vi "Short-Term Flicker Severity.vi"(0 "Pinst":waveform(dbl)[](array[waveform]), 1 "reset? (F)":bool, 9 "system info in":refnum<class "EP System Info.lvclass">, 11 "error in (no error)":errorcluster) -> (4 "Pst":dbl[](array[numeric]), 6 "Pst timestamp":timestamp, 10 "system info out":refnum<class "EP System Info.lvclass">, 14 "output valid?":bool, 15 "error out":errorcluster)   [LabVIEW 2014, in "NI_EP_Power Quality.lvlib"]
doc: "Aggregates instantaneous flicker values and returns the short-term flicker of a voltage waveform for a 10-minute period, according to IEC 61000-4-15:2010.\n\nThis VI supports measuring single-bus single-line or multiple-bus single-line systems."
uses:
  <vilib>/addons/Electrical Power/PQ/NI_EP_Power Quality.lvlib
  <vilib>/addons/Electrical Power/PQ/Common/Classes/System Info/EP System Info.lvclass
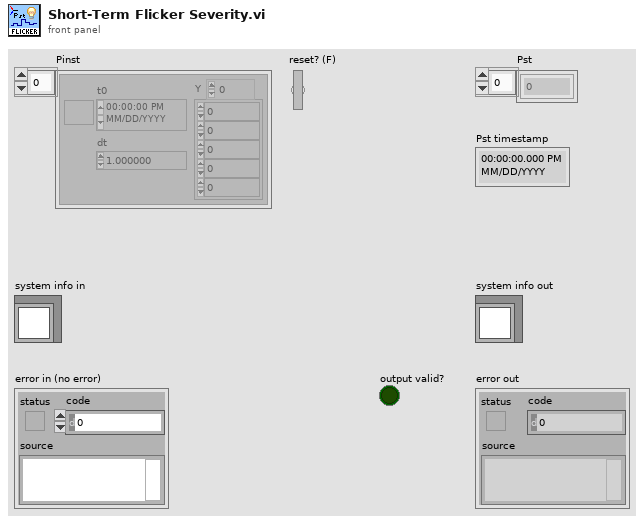
[diagram p1: front panel]
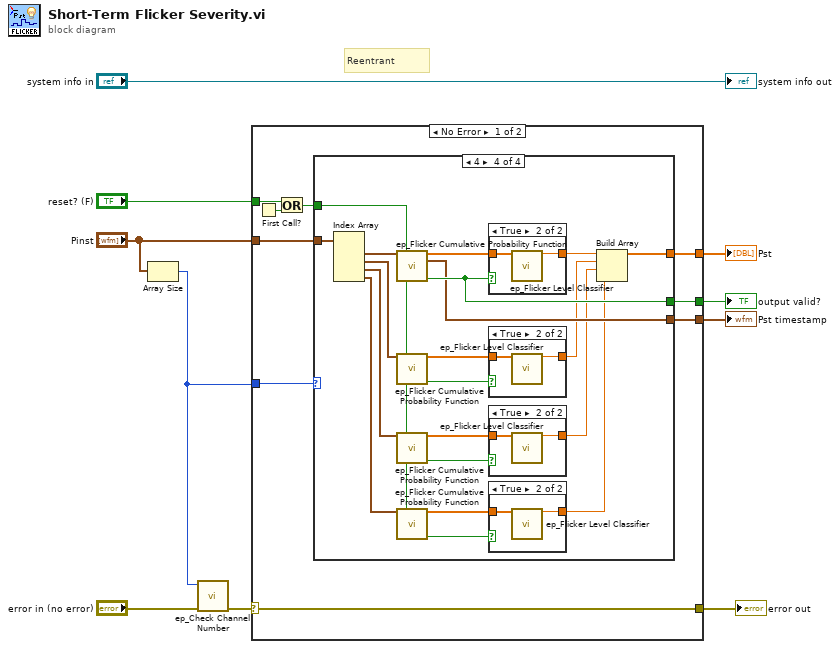
[diagram p0: block diagram]
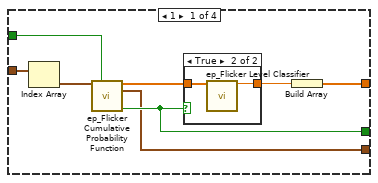
[diagram p2: hidden frame]
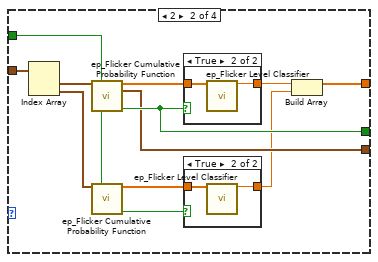
[diagram p4: hidden frame]
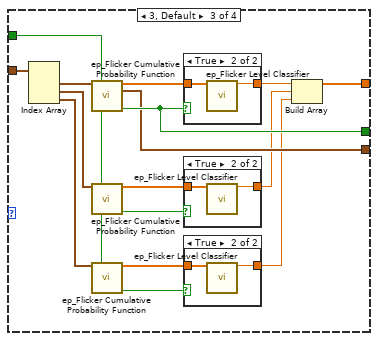
[diagram p7: hidden frame]
diagram:
  # "Reentrant"
  n1 = Array Size(array="Pinst") -> (size(s)=w3:i32)
  n2 = call <vilib>:"ep_Check Channel Number.vi"("channel number"=w3, "error in (no error)"="error in (no error)") -> ("error out"=w2:errorcluster)  [unwired: 13 in]
  n3 = case shown="No Error" w2 {
    selector: w2 -> [w11 w96]
    tunnel: [w19 _] -> w10
    tunnel: [w18 _] -> w9
    tunnel: [w17 _] -> w8
    tunnel: "reset? (F)" -> [w16 _]
    tunnel: "Pinst" -> [w15 _]
    tunnel: w3 -> [w12 _]
    tunnel: [w11 w96] -> w1
    frame No Error {
      n4 = First Call?() -> (First Call?: T/F=w14:bool)
      n5 = Or(x=w16, y=w14) -> (x .or. y?=w13:bool)
      n6 = case shown="4" w12 {
        tunnel: w15 -> [w27 w41 w61 w87]
        tunnel: w13 -> [w25 w38 w57 w69]
        tunnel: [w22 w34 w53 w80] -> w19
        tunnel: [w21 w35 w54 w81] -> w18
        tunnel: [w20 w33 w52 w79] -> w17
        frame 1 {
          n7 = Index Array(array=w27) -> (element=w26:waveform(dbl))  [unwired: 1 in]
          n8 = call <vilib>:"ep_Flicker Cumulative Probability Function.vi"("instantaneous flicker Pinst (Output 5)"=w26, "restart (F)"=w25) -> ("flicker cumulative probability function"=w24:dbl[], "Pst flicker time"=w20:timestamp, "data valid?"=w21:bool)  [unwired: 11 in]
          n9 = case shown="True" w21 {
            tunnel: w24 -> [_ w29]
            tunnel: [_ w28] -> w23
            frame False {
            }
            frame True {
              n10 = call <vilib>:"ep_Flicker Level Classifier.vi"("flicker cumulative probability function"=w29) -> ("flicker Pst"=w28:dbl)  [unwired: 14 in]
            }
          }
          n11 = Build Array(w23) -> (w22:dbl[])
        }
        frame 2 {
          n12 = Index Array(array=w41) -> (element #1=w40:waveform(dbl), element #2=w39:waveform(dbl))  [unwired: 2 in]
          n13 = call <vilib>:"ep_Flicker Cumulative Probability Function.vi"("instantaneous flicker Pinst (Output 5)"=w40, "restart (F)"=w38) -> ("flicker cumulative probability function"=w36:dbl[], "Pst flicker time"=w33:timestamp, "data valid?"=w35:bool)  [unwired: 11 in]
          n14 = call <vilib>:"ep_Flicker Cumulative Probability Function.vi"("instantaneous flicker Pinst (Output 5)"=w39, "restart (F)"=w38) -> ("flicker cumulative probability function"=w32:dbl[], "data valid?"=w31:bool)  [unwired: 11 in, 1 out]
          n15 = case shown="True" w35 {
            tunnel: w36 -> [_ w45]
            tunnel: [_ w44] -> w37
            frame False {
            }
            frame True {
              n16 = call <vilib>:"ep_Flicker Level Classifier.vi"("flicker cumulative probability function"=w45) -> ("flicker Pst"=w44:dbl)  [unwired: 14 in]
            }
          }
          n17 = case shown="True" w31 {
            tunnel: w32 -> [_ w43]
            tunnel: [_ w42] -> w30
            frame False {
            }
            frame True {
              n18 = call <vilib>:"ep_Flicker Level Classifier.vi"("flicker cumulative probability function"=w43) -> ("flicker Pst"=w42:dbl)  [unwired: 14 in]
            }
          }
          n19 = Build Array(w37, w30) -> (w34:dbl[])
        }
        frame 3, Default {
          n20 = Index Array(array=w61) -> (element #1=w60:waveform(dbl), element #2=w59:waveform(dbl), element #3=w58:waveform(dbl))  [unwired: 3 in]
          n21 = call <vilib>:"ep_Flicker Cumulative Probability Function.vi"("instantaneous flicker Pinst (Output 5)"=w60, "restart (F)"=w57) -> ("flicker cumulative probability function"=w55:dbl[], "Pst flicker time"=w52:timestamp, "data valid?"=w54:bool)  [unwired: 11 in]
          n22 = call <vilib>:"ep_Flicker Cumulative Probability Function.vi"("instantaneous flicker Pinst (Output 5)"=w59, "restart (F)"=w57) -> ("flicker cumulative probability function"=w51:dbl[], "data valid?"=w49:bool)  [unwired: 11 in, 1 out]
          n23 = call <vilib>:"ep_Flicker Cumulative Probability Function.vi"("instantaneous flicker Pinst (Output 5)"=w58, "restart (F)"=w57) -> ("flicker cumulative probability function"=w50:dbl[], "data valid?"=w48:bool)  [unwired: 11 in, 1 out]
          n24 = case shown="True" w54 {
            tunnel: w55 -> [_ w67]
            tunnel: [_ w66] -> w56
            frame False {
            }
            frame True {
              n25 = call <vilib>:"ep_Flicker Level Classifier.vi"("flicker cumulative probability function"=w67) -> ("flicker Pst"=w66:dbl)  [unwired: 14 in]
            }
          }
          n26 = case shown="True" w49 {
            tunnel: w51 -> [_ w65]
            tunnel: [_ w64] -> w47
            frame False {
            }
            frame True {
              n27 = call <vilib>:"ep_Flicker Level Classifier.vi"("flicker cumulative probability function"=w65) -> ("flicker Pst"=w64:dbl)  [unwired: 14 in]
            }
          }
          n28 = case shown="True" w48 {
            tunnel: w50 -> [_ w63]
            tunnel: [_ w62] -> w46
            frame False {
            }
            frame True {
              n29 = call <vilib>:"ep_Flicker Level Classifier.vi"("flicker cumulative probability function"=w63) -> ("flicker Pst"=w62:dbl)  [unwired: 14 in]
            }
          }
          n30 = Build Array(w56, w47, w46) -> (w53:dbl[])
        }
        frame 4 {
          n31 = Index Array(array=w87) -> (element #1=w86:waveform(dbl), element #2=w85:waveform(dbl), element #3=w84:waveform(dbl), element #4=w70:waveform(dbl))  [unwired: 4 in]
          n32 = call <vilib>:"ep_Flicker Cumulative Probability Function.vi"("instantaneous flicker Pinst (Output 5)"=w86, "restart (F)"=w69) -> ("flicker cumulative probability function"=w82:dbl[], "Pst flicker time"=w79:timestamp, "data valid?"=w81:bool)  [unwired: 11 in]
          n33 = call <vilib>:"ep_Flicker Cumulative Probability Function.vi"("instantaneous flicker Pinst (Output 5)"=w85, "restart (F)"=w69) -> ("flicker cumulative probability function"=w78:dbl[], "data valid?"=w76:bool)  [unwired: 11 in, 1 out]
          n34 = call <vilib>:"ep_Flicker Cumulative Probability Function.vi"("instantaneous flicker Pinst (Output 5)"=w84, "restart (F)"=w69) -> ("flicker cumulative probability function"=w77:dbl[], "data valid?"=w75:bool)  [unwired: 11 in, 1 out]
          n35 = call <vilib>:"ep_Flicker Cumulative Probability Function.vi"("instantaneous flicker Pinst (Output 5)"=w70, "restart (F)"=w69) -> ("flicker cumulative probability function"=w71:dbl[], "data valid?"=w72:bool)  [unwired: 11 in, 1 out]
          n36 = case shown="True" w81 {
            tunnel: w82 -> [_ w95]
            tunnel: [_ w94] -> w83
            frame False {
            }
            frame True {
              n37 = call <vilib>:"ep_Flicker Level Classifier.vi"("flicker cumulative probability function"=w95) -> ("flicker Pst"=w94:dbl)  [unwired: 14 in]
            }
          }
          n38 = case shown="True" w76 {
            tunnel: w78 -> [_ w93]
            tunnel: [_ w92] -> w74
            frame False {
            }
            frame True {
              n39 = call <vilib>:"ep_Flicker Level Classifier.vi"("flicker cumulative probability function"=w93) -> ("flicker Pst"=w92:dbl)  [unwired: 14 in]
            }
          }
          n40 = case shown="True" w75 {
            tunnel: w77 -> [_ w91]
            tunnel: [_ w90] -> w73
            frame False {
            }
            frame True {
              n41 = call <vilib>:"ep_Flicker Level Classifier.vi"("flicker cumulative probability function"=w91) -> ("flicker Pst"=w90:dbl)  [unwired: 14 in]
            }
          }
          n42 = case shown="True" w72 {
            tunnel: w71 -> [_ w89]
            tunnel: [_ w88] -> w68
            frame False {
            }
            frame True {
              n43 = call <vilib>:"ep_Flicker Level Classifier.vi"("flicker cumulative probability function"=w89) -> ("flicker Pst"=w88:dbl)  [unwired: 14 in]
            }
          }
          n44 = Build Array(w83, w74, w73, w68) -> (w80:dbl[])
        }
      }
    }
    frame Error {
    }
  }
  "error out" <- w1
  "Pst" <- w10
  "output valid?" <- w9
  "Pst timestamp" <- w8
  "system info out" <- "system info in"
